vi "EnvSensors.vi"() -> ()   [LabVIEW 2016]
uses:
  iowkit.dll
panel:
  out "Environmental data":cluster{timestamp[], sgl[]}[](graph)
  in  "Start/stop acquisition":bool
  in  "stop":bool
  out "Sensor status":bool
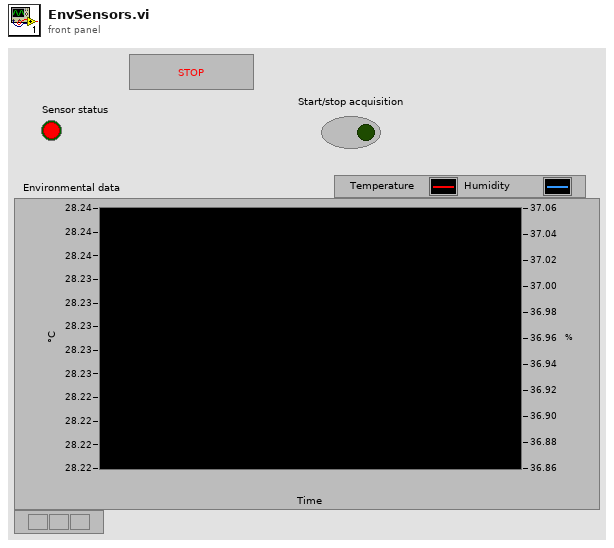
[diagram p1: front panel]
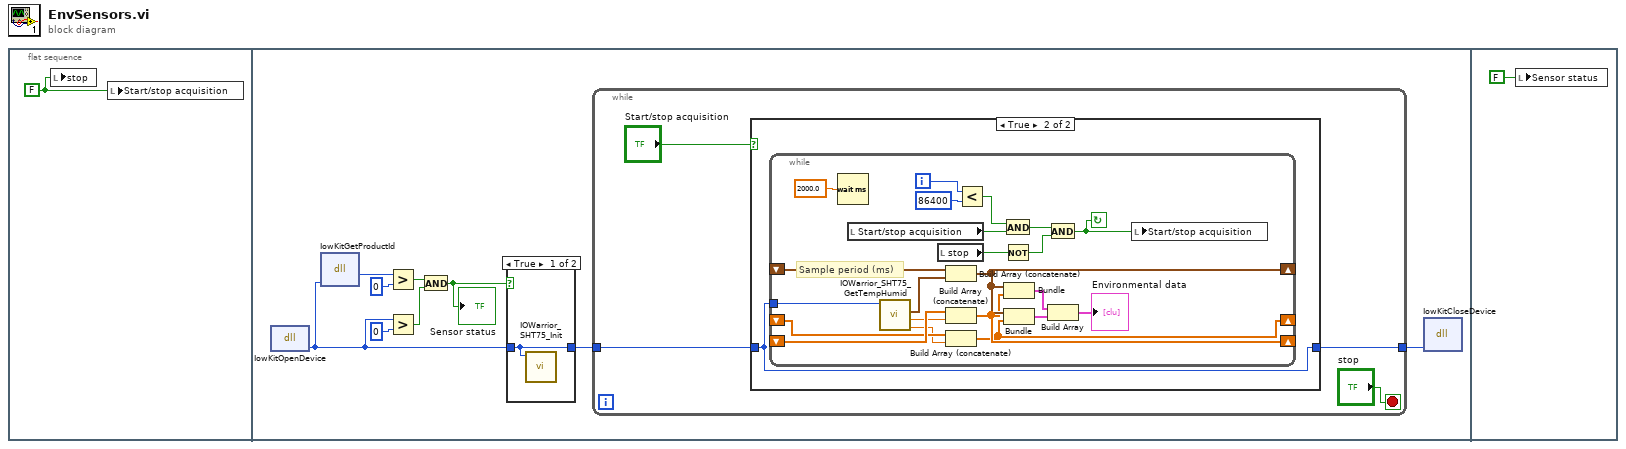
[diagram p0: block diagram]
diagram:
  n1 = flat-sequence {
    frame #0 {
      w1 = FALSE
      n2 = local write "stop"(w1) -> ()
      n3 = local write "Start/stop acquisition"(w1) -> ()
    }
    frame #1 {
      n4 = dll-call lib="C:/Users/Administrator/Desktop/HGCAL_sensor_tests/iowkit.dll" fn="IowKitOpenDevice"() -> ("return type"=w10:i64)  [unwired: 3 in, 2 out]
      n5 = dll-call lib="C:/Users/Administrator/Desktop/HGCAL_sensor_tests/iowkit.dll" fn="IowKitGetProductId"("devHandle"=w10) -> ("prodID"=w6:u16)  [unwired: 3 in, 3 out]
      n6 = Greater?(x=w6, y=0) -> (0:w9:bool)
      n7 = Greater?(x=w10, y=0) -> (0:w8:bool)
      n8 = And(x=w9, y=w8) -> (x .and. y?=w7:bool)
      "Sensor status" <- w7
      n9 = case shown="True" w7 {
        tunnel: w10 -> [w11 w12]
        tunnel: [w11 w12] -> w2
        frame True {
          n10 = call "IOWarrior_SHT75_Init.vi"("Dongle handle"=w11) -> ()  [unwired: 11 out]
        }
        frame False {
        }
      }
      n11 = while {
        tunnel: w2 -> [w15]
        tunnel: [w13] -> w3
        stop <- "stop" stop-if-true
        n12 = case shown="True" "Start/stop acquisition" {
          tunnel: w15 -> [w17 w18]
          tunnel: [w17 w18] -> w13
          frame False {
          }
          frame True {
            n13 = while {
              tunnel: w18 -> [w32]
              shift-right: [w23] -> _
              shift-left: _ -> [w28]
              shift-right: [w22] -> _
              shift-left: _ -> [w27]
              shift-right: [w24] -> _
              shift-left: _ -> [w26]
              i -> [w34]
              stop <- w33 continue-if-true
              # "Sample period (ms)"
              n14 = Wait (ms)(milliseconds to wait=sgl 2000.0 ("Sample period (s)")) -> ()  [unwired: 1 out]
              n15 = local read "Start/stop acquisition"() -> (w37:bool)
              n16 = call "IOWarrior_SHT75_GetTempHumid.vi"("Dongle handle"=w32) -> ("Humidity"=w20:sgl, "Temperature"=w21:sgl, "Time Stamp"=w29:timestamp)  [unwired: 7 out]
              n17 = local read "stop"() -> (w40:bool)
              n18 = Build Array (concatenate)(w26, w29) -> (w24:timestamp[])
              n19 = Build Array (concatenate)(w28, w21) -> (w23:sgl[])
              n20 = Build Array (concatenate)(w27, w20) -> (w22:sgl[])
              n21 = Less?(x=w34, y=86400) -> (x < y?=w36:bool)
              n22 = And(x=w36, y=w37) -> (x .and. y?=w38:bool)
              n23 = Not(x=w40) -> (.not. x?=w39:bool)
              n24 = Bundle(w24, w23) -> (w31:cluster{timestamp[], sgl[]})  [unwired: 1 out]
              n25 = Bundle(w24, w22) -> (w30:cluster{timestamp[], sgl[]})  [unwired: 1 out]
              n26 = And(x=w38, y=w39) -> (x .and. y?=w33:bool)
              n27 = Build Array(w31, w30) -> (→"Environmental data":cluster{timestamp[], sgl[]}[])
              n28 = local write "Start/stop acquisition"(w33) -> ()
            }
          }
        }
      }
      n29 = dll-call lib="C:/Users/Administrator/Desktop/HGCAL_sensor_tests/iowkit.dll" fn="IowKitCloseDevice"("devHandle"=w3) -> ()  [unwired: 3 in, 4 out]
    }
    frame #2 {
      n30 = local write "Sensor status"(FALSE) -> ()
    }
  }
